vi "Sound Out.vi"(8 "error in (no error)":errorcluster, 10 "sampling info":cluster{"Fs":dbl, "#s":dbl}={"Fs"=22050.0, "#s"=220500.0}, 11 "Detected Frequency (Hz)":dbl) -> (0 "error out":errorcluster, 3 "task ID out":T1 format="%.0x")   [LabVIEW 2018, in "CollectionSupport.lvlib"]
uses:
  CollectionSupport.lvlib
  <vilib>/sound2/lvsound2.llb/Sound Output Task ID.ctl
  <vilib>/sound2/lvsound2.llb/Sound Output Write (DBL Single).vi
  <vilib>/measure/NI_MABase.lvlib
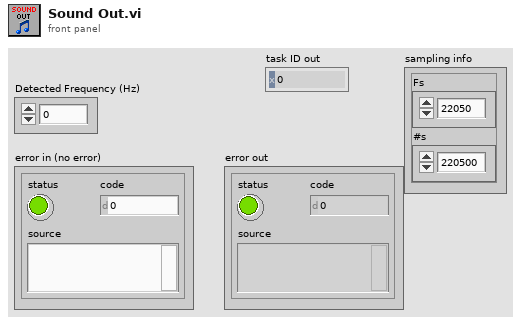
[diagram p1: front panel]
types:
  T1 = typedef "Sound Output Task ID.ctl" = u32
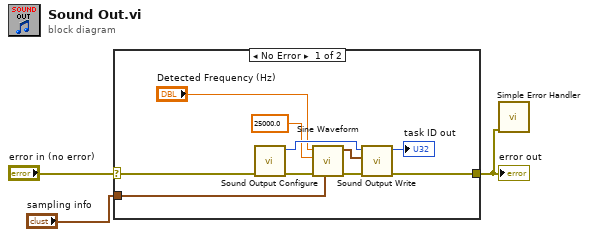
[diagram p0: block diagram]
diagram:
  n1 = case shown="No Error" "error in (no error)" {
    selector: "error in (no error)" -> [w13 w14]
    tunnel: [w10 w14] -> w2
    tunnel: "sampling info" -> [w5 _]
    frame No Error {
      n2 = call <vilib>:"Sound Output Configure.vi"("error in (no error)"=w13) -> ("error out"=w12:errorcluster, "task ID"=w9:T1)  [unwired: 9 in]
      n3 = call <vilib>:"Sine Waveform.vi"("sampling info"=w5, "error in (no error)"=w12, "amplitude"=25000.0, "frequency"="Detected Frequency (Hz)") -> ("error out"=w11:errorcluster, "signal out"=w6:waveform(dbl))  [unwired: 6 in]
      n4 = call-poly <vilib>:"Sound Output Write.vi"("error in (no error)"=w11, "data"=w6, "task ID"=w9) -> ("error out"=w10:errorcluster, "task ID out"=→"task ID out":T1)  [unwired: 7 in]
    }
    frame Error {
    }
  }
  "error out" <- w2
  n5 = call <vilib>:"Simple Error Handler.vi"("error in (no error)"=w2) -> ()  [unwired: 4 in, 5 out]
